vi "create default alias.vi"(8 "error in":errorcluster, 11 "configuration in":refnum<class "Bus Configuration.lvclass">) -> (0 "error out":errorcluster, 2 "default alias":string, 3 "configuration out":refnum<class "Bus Configuration.lvclass">)   [LabVIEW 2014, in "Bus Configuration.lvclass"]
uses:
  Bus Configuration.lvclass
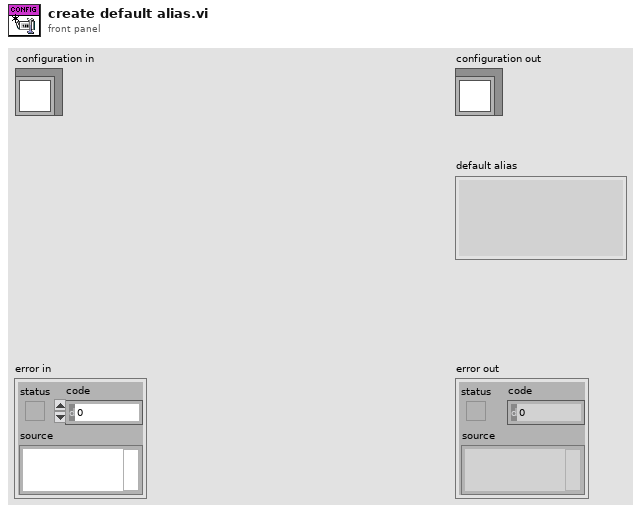
[diagram p1: front panel]
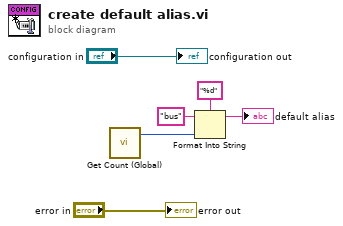
[diagram p0: block diagram]
diagram:
  n1 = call "Get Count (Global).vi"() -> ("Count"=w2:u32)  [unwired: 11 in]
  n2 = Format Into String(format string="%d", initial string="bus" ("default alias"), w2) -> (resulting string=→"default alias":string)  [unwired: 1 in, 1 out]
  "error out" <- "error in"
  "configuration out" <- "configuration in"
